vi "DAC Configure FP View.vi"(8 "error in":errorcluster, 11 "DAC Keller Diff P 23X in":refnum<class "DAC Keller Diff P 23X.lvclass">) -> (0 "error out":errorcluster, 3 "DAC Keller Diff P 23X out":refnum<class "DAC Keller Diff P 23X.lvclass">)   [LabVIEW 2019, in "DAC.lvlib" / "DAC Keller Diff P 23X.lvclass"]
uses:
  DAC Keller Diff P 23X.lvclass
  C:/Users/wg/Documents/LV_Projects/test-stand/App/DAC/DAC.lvclass
  Results/Results Method.ctl
  Results/DeepU Results/DeepU Results.lvclass
  DAC.lvclass/DAC.ctl
  DAC Keller Diff P 23X.lvclass/DAC Keller Diff P 23X.ctl
  Results/Results.lvlib
  DAC.lvclass
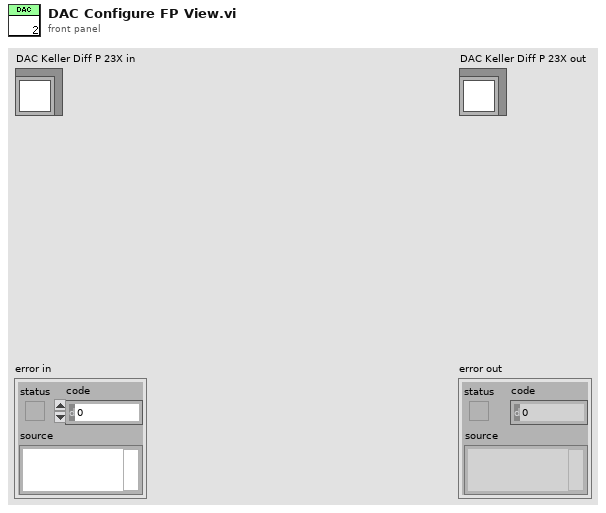
[diagram p1: front panel]
types:
  T1 = typedef "Results.lvlib/Results Method.ctl" = enum16{"Get", "Set"}
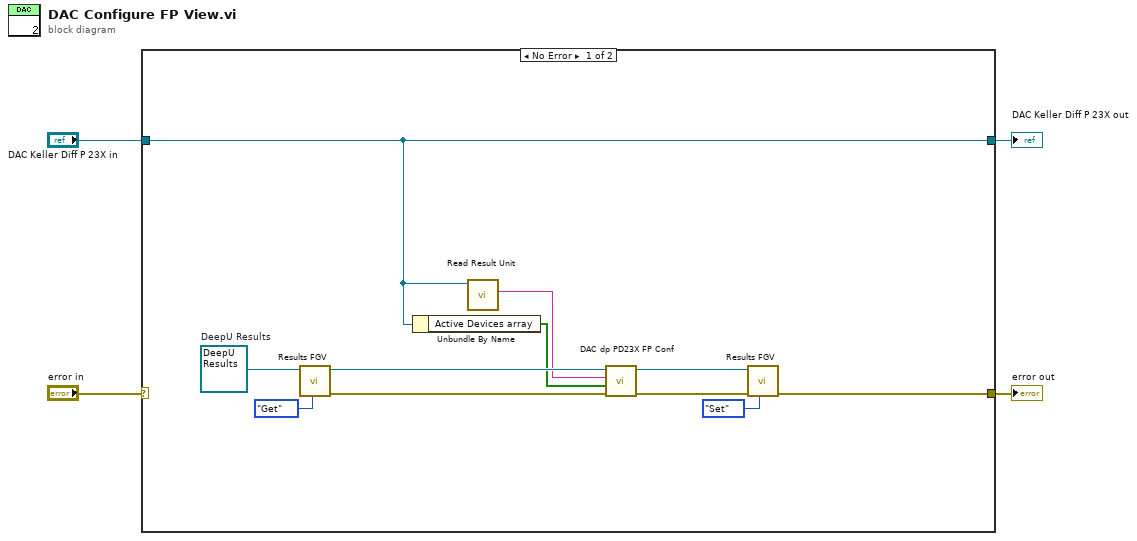
[diagram p0: block diagram]
diagram:
  n1 = case shown="No Error" "error in" {
    selector: "error in" -> [_ w17]
    tunnel: [w15 w17] -> w1
    tunnel: [w14 w16] -> w2
    tunnel: "DAC Keller Diff P 23X in" -> [w14 w16]
    frame No Error {
      w13 = refnum<class "DeepU Results.lvclass"> refnum  # DeepU Results
      n2 = call-dynamic "Results FGV.vi"("Method"=Results_Method."Get", "DeepU Results in"=w13) -> ("error out"=w8:errorcluster, "DeepU Results out"=w10:refnum<class "DeepU Results.lvclass">)  [unwired: 8 in]
      n3 = Unbundle By Name(w14) -> ("Active Devices array"=w5:bool[])
      n4 = call "Read Result Unit.vi"("DAC in"=w14) -> ("Unit"=w6:string)  [unwired: 8 in, 2 out]
      n5 = call "DAC dp PD23X FP Conf.vi"("error in (no error)"=w8, "Used dp PD23X"=w5, "Result Unit"=w6, "DeepU Results in"=w10) -> ("error out"=w7:errorcluster, "DeepU Results out"=w9:refnum<class "DeepU Results.lvclass">)  [unwired: 6 in]
      n6 = call-dynamic "Results FGV.vi"("Method"=Results_Method."Set", "error in"=w7, "DeepU Results in"=w9) -> ("error out"=w15:errorcluster)  [unwired: 7 in, 1 out]
    }
    frame Error {
    }
  }
  "error out" <- w1
  "DAC Keller Diff P 23X out" <- w2
